vi "反控交互.vi"() -> ()   [LabVIEW 2016, in "质控单元V4.lvlib"]
panel:
  in  "启动参数":T1
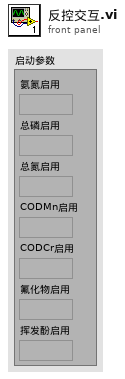
[diagram p1: front panel]
types:
  T1 = typedef "质控单元V4.lvlib/启动参数.ctl" = cluster{"氨氮启用":bool, "总磷启用":bool, "总氮启用":bool, "CODMn启用":bool, "CODCr启用":bool, "氟化物启用":bool, "挥发酚启用":bool}
  T2 = typedef "质控单元V4.lvlib/数据流类型.ctl" = cluster{"cmd":enum16{"start", "stop"}, "data":variant}
  T3 = typedef "质控单元V4.lvlib/测试流程.ctl" = enum16{"加标回收（启动采配水）", "加标回收（不启动采配水）", "水样测试（启动采配水）", "水样测试（不启动采配水）", "平行样测试（启动采配水）", "平行样测试（不启动采配水）", "集成干预测试"}
  T4 = typedef "质控slave id.ctl" = enum16{"null", "氨氮", "总磷", "总氮", "CODMn", "CODCr", "氟化物"}
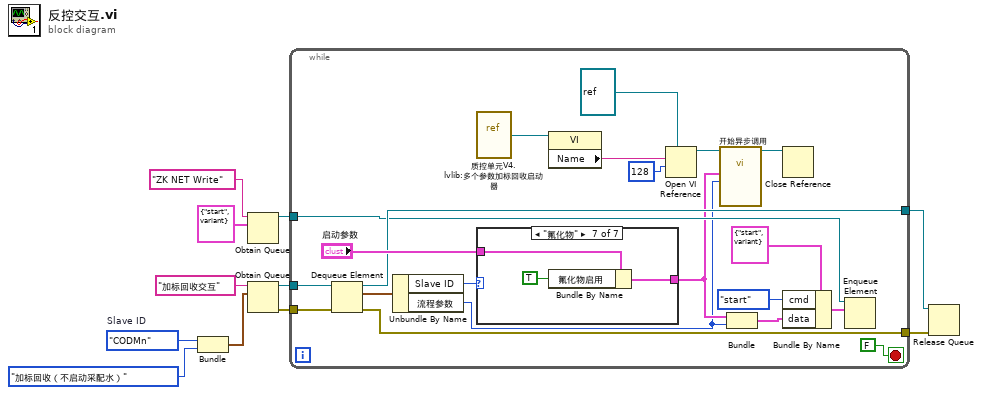
[diagram p0: block diagram]
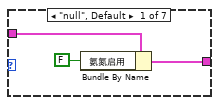
[diagram p2: hidden frame]
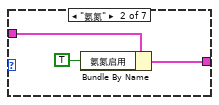
[diagram p3: hidden frame]
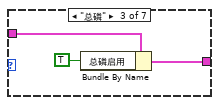
[diagram p4: hidden frame]
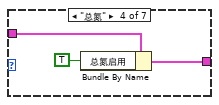
[diagram p5: hidden frame]
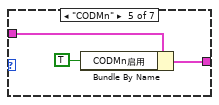
[diagram p6: hidden frame]
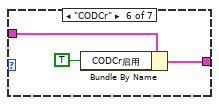
[diagram p7: hidden frame]
diagram:
  w8 = 质控slave_id."CODMn"  # Slave ID
  n1 = Bundle("Slave ID"=w8, "流程参数"=测试流程."加标回收（不启动采配水）") -> (w7:cluster{"Slave ID":T4, "流程参数":T3})  [unwired: 1 in]
  n2 = Obtain Queue(name (unnamed)="ZK NET Write" ("名称（未命名）"), element data type=T2 {"cmd"=enum."start", "data"=variant} ("簇")) -> (queue out=w1:refnum<queue>)  [unwired: 3 in, 2 out]
  n3 = Obtain Queue(name (unnamed)="加标回收交互" ("名称（未命名）"), element data type=w7) -> (queue out=w11:refnum<queue>, error out=w10:errorcluster)  [unwired: 3 in, 1 out]
  n4 = while {
    tunnel: w11 -> [w32]
    tunnel: w10 -> [w31]
    tunnel: [w20] -> w5
    tunnel: [w19] -> w4
    tunnel: w1 -> [w15]
    stop <- FALSE stop-if-true
    n5 = Dequeue Element(queue=w32, error in (no error)=w31) -> (queue out=w20:refnum<queue>, element=w29:cluster{"Slave ID":T4, "流程参数":T3}, error out=w19:errorcluster)  [unwired: 1 in, 1 out]
    n6 = Unbundle By Name(w29) -> ("Slave ID"=w22:T4, "流程参数"=w13:T3)
    n7 = vi-ref "质控单元V4.lvlib:多个参数加标回收启动器.vi"() -> (w28:refnum<vi>)
    n8 = case shown="\"氟化物\"" w22 {
      tunnel: "启动参数" -> [w34 w38 w40 w43 w46 w49 w52]
      tunnel: [w33 w36 w39 w42 w45 w48 w51] -> w14
      frame "null", Default {
        n9 = Bundle By Name(cluster=w34, "氨氮启用"=FALSE) -> (w33:T1)
      }
      frame "氨氮" {
        n10 = Bundle By Name(cluster=w38, "氨氮启用"=TRUE) -> (w36:T1)
      }
      frame "总磷" {
        n11 = Bundle By Name(cluster=w40, "总磷启用"=TRUE ("氨氮启用")) -> (w39:T1)
      }
      frame "总氮" {
        n12 = Bundle By Name(cluster=w43, "总氮启用"=TRUE ("氨氮启用")) -> (w42:T1)
      }
      frame "CODMn" {
        n13 = Bundle By Name(cluster=w46, "CODMn启用"=TRUE ("氨氮启用")) -> (w45:T1)
      }
      frame "CODCr" {
        n14 = Bundle By Name(cluster=w49, "CODCr启用"=TRUE ("氨氮启用")) -> (w48:T1)
      }
      frame "氟化物" {
        n15 = Bundle By Name(cluster=w52, "氟化物启用"=TRUE ("氨氮启用")) -> (w51:T1)
      }
    }
    n16 = property class="VI"(reference=w28) -> ("Name"=w27:string)  [unwired: 1 in, 2 out]
    n17 = Open VI Reference(type specifier VI Refnum (for type only)=refnum<vi> refnum, vi path=w27, options=128 ("选项")) -> (vi reference=w25:refnum<vi>)  [unwired: 3 in, 1 out]
    n18 = call-by-ref "开始异步调用"(reference=w25, "流程"=w13, "启用参数选择"=w14) -> (reference out=w24:refnum<vi>)  [unwired: 11 in, 1 out]
    n19 = Bundle("启动参数"=w14, "流程参数"=w13) -> (w12:cluster{"启动参数":T1, "流程参数":T3})  [unwired: 1 in]
    n20 = Close Reference(reference=w24) -> ()  [unwired: 1 in, 1 out]
    n21 = Bundle By Name(cluster=T2 {"cmd"=enum."start", "data"=variant} ("簇"), "cmd"=enum16{"start", "stop"}."start", "data"=w12) -> (w16:T2)
    n22 = Enqueue Element(queue=w15, element=w16) -> ()  [unwired: 2 in, 3 out]
  }
  n23 = Release Queue(queue=w5, error in (no error)=w4) -> ()  [unwired: 1 in, 3 out]
